vi "CreateDateNamedDirectory.vi"(2 "error in":errorcluster, 3 "base path":path=path "c:/") -> (0 "error out":errorcluster, 1 "created path":path)   [LabVIEW 2014]
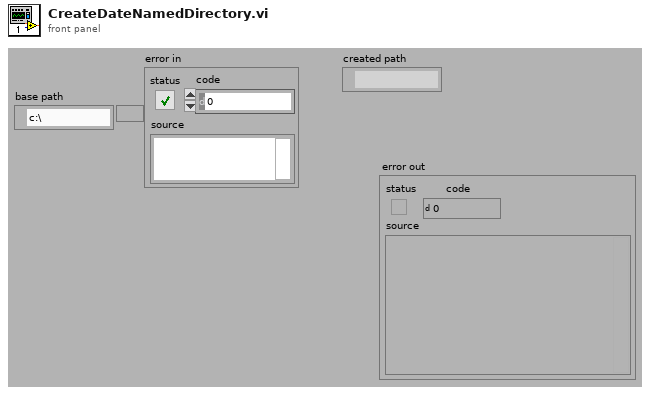
[diagram p1: front panel]
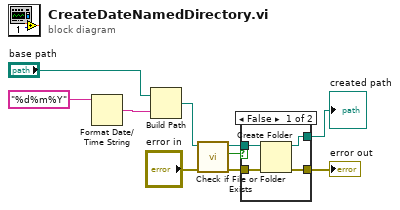
[diagram p0: block diagram]
diagram:
  n1 = Format Date/Time String(time format string (%c)="%d%m%Y") -> (date/time string=w9:string)  [unwired: 2 in]
  n2 = Build Path(base path="base path", name or relative path=w9) -> (appended path=w6:path)
  n3 = call <vilib>:"Check if File or Folder Exists.vi"("error in (no error)"="error in", "path"=w6) -> ("error out"=w3:errorcluster, "file or folder exists?"=w5:bool, "dup path"=w4:path)  [unwired: 7 in]
  n4 = case shown="False" w5 {
    tunnel: w4 -> [w14 w15]
    tunnel: [w13 w16] -> w2
    tunnel: w3 -> [w12 w16]
    tunnel: [w11 w15] -> w1
    frame False {
      n5 = Create Folder(path (use dialog)=w14, error in=w12) -> (created path=w11:path, error out=w13:errorcluster)  [unwired: 1 in, 1 out]
    }
    frame True {
    }
  }
  "created path" <- w1
  "error out" <- w2
